vi "Read Path Refnum.vi"(8 "error in (no error)":errorcluster, 11 "Path Control in":refnum<class "Path Control.lvclass">) -> (0 "error out":errorcluster, 2 "Path Refnum":refnum<vi>, 3 "Path Control out":refnum<class "Path Control.lvclass">)   [LabVIEW 2010, in "Path Control.lvclass"]
uses:
  Path Control.lvclass
  Path Control.lvclass/Path Control.ctl
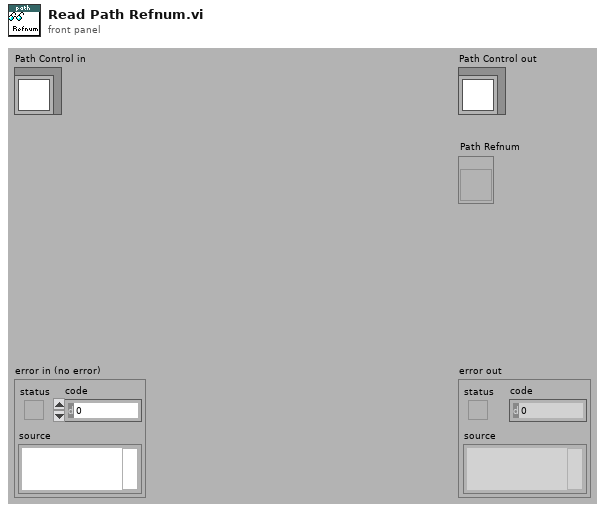
[diagram p1: front panel]
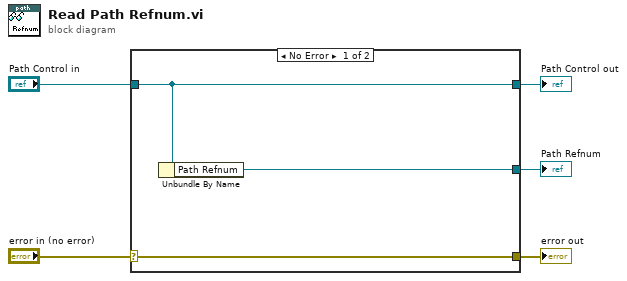
[diagram p0: block diagram]
diagram:
  n1 = case shown="No Error" "error in (no error)" {
    selector: "error in (no error)" -> [w8 w9]
    tunnel: [w8 w9] -> w4
    tunnel: [w7 w10] -> w2
    tunnel: "Path Control in" -> [w7 w10]
    tunnel: [w6 _] -> w1
    frame No Error {
      n2 = Unbundle By Name(w7) -> ("Path Refnum"=w6:refnum<vi>)
    }
    frame Error {
    }
  }
  "error out" <- w4
  "Path Control out" <- w2
  "Path Refnum" <- w1
